vi "Shutdown.vi"(10 "Boiler Simulation Controls":T1 {"Flame Sensor Value (%)" min=0.0 max=100.0 scale=0.0..100.0}, 11 "Boiler Controls":T2 {"Fuel Valve Position" min=0.0 max=100.0 scale=0.0..100.0 scale format="%.2f"}) -> (3 "result":bool)   [LabVIEW 2015]
uses:
  USB Template (LV 8.6)/Boiler/Controls/Boiler Controls.ctl
  USB Template (LV 8.6)/Boiler/Controls/Boiler Simulation Controls.ctl
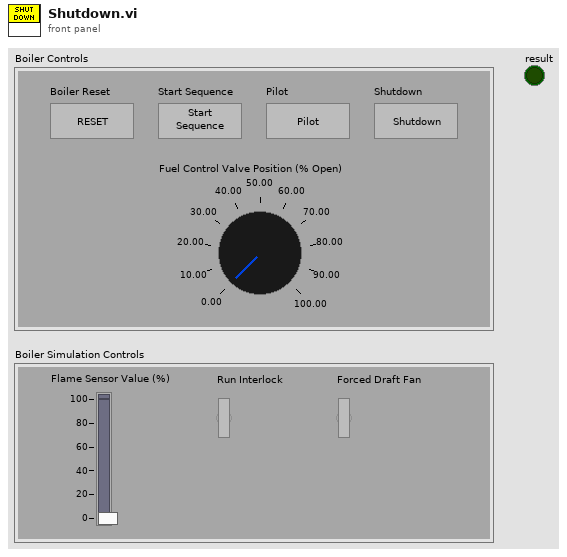
[diagram p1: front panel]
types:
  T1 = typedef "Boiler Simulation Controls.ctl" = cluster{"Flame Sensor Value (%)":dbl, "Run Interlock":bool, "Forced Draft Fan":bool}
  T2 = typedef "Boiler Controls.ctl" = cluster{"Boiler Reset":bool, "Start Sequence":bool, "Pilot":bool, "Shutdown":bool, "Fuel Valve Position":dbl}
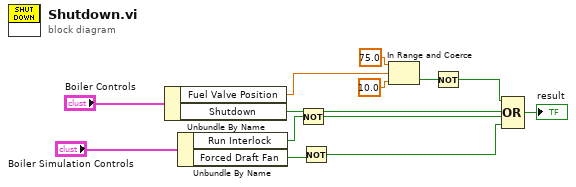
[diagram p0: block diagram]
diagram:
  n1 = Unbundle By Name("Boiler Controls") -> ("Fuel Valve Position"=w5:dbl, "Shutdown"=w11:bool)
  n2 = Unbundle By Name("Boiler Simulation Controls") -> ("Run Interlock"=w10:bool, "Forced Draft Fan"=w8:bool)
  n3 = Not(x=w10) -> (.not. x?=w1:bool)
  n4 = Not(x=w8) -> (.not. x?=w9:bool)
  n5 = In Range and Coerce(upper limit=75.0, x=w5, lower limit=10.0) -> (In Range?=w6:bool)  [unwired: 1 out]
  n6 = Not(x=w6) -> (.not. x?=w12:bool)
  n7 = Compound Arithmetic op=OR(w12, w11, w1, w9) -> (→"result":bool)
